vi "Motor sequence -- FGV.vi"(7 "Motor params":T2, 8 "error in (no error)":errorcluster, 10 "current position (in)":dbl, 11 "Action":T1=enum."Full step") -> (0 "error out":errorcluster, 3 "Data out":bool[](array[boolean]), 5 "current position (out)":dbl)   [LabVIEW 2020, in "GUI.lvlib"]
uses:
  GUI.lvlib
  <userlib>/_OpenG.lib/array/array.llb/openg_array.lvlib
  <userlib>/_OpenG.lib/array/array.llb/Reverse 2D Array (Boolean)__ogtk.vi
  Support/Motor parameters.ctl
  FGV states.ctl
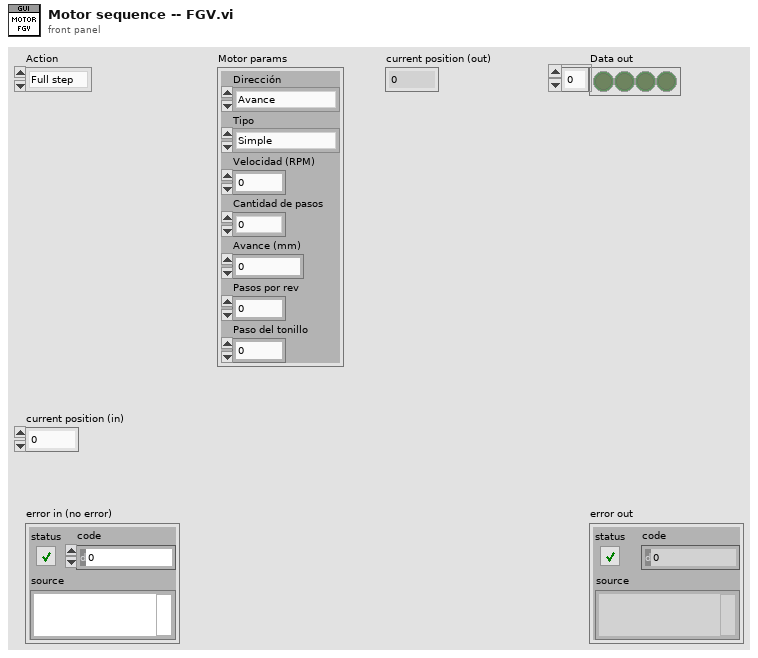
[diagram p1: front panel]
types:
  T1 = typedef "GUI.lvlib/FGV states.ctl" = enum16{"Read", "Full step", "Half step", "Release", "Reset"}
  T2 = typedef "GUI.lvlib/Motor parameters.ctl" = cluster{"Dirección":enum16{"Avance", "Retroceso"}, "Tipo":enum16{"Simple", "Medio paso"}, "Velocidad (RPM)":dbl, "Cantidad de pasos":i32, "Avance (mm)":dbl, "Pasos por rev":dbl, "Paso del tonillo":dbl}
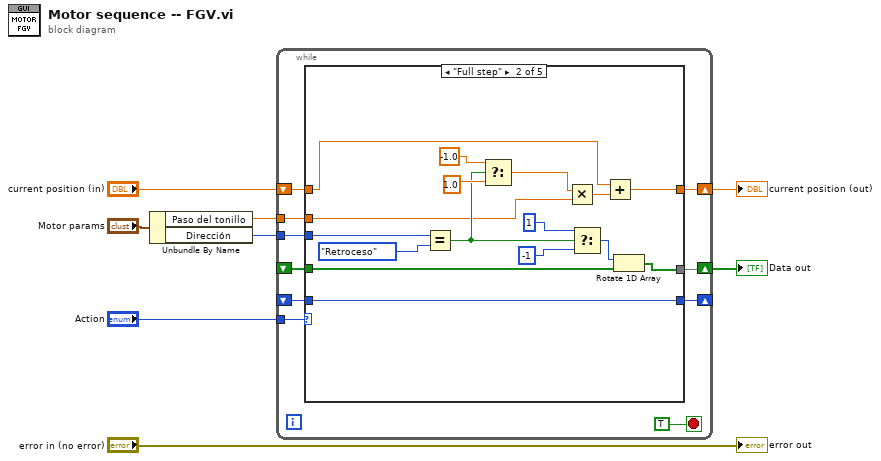
[diagram p0: block diagram]
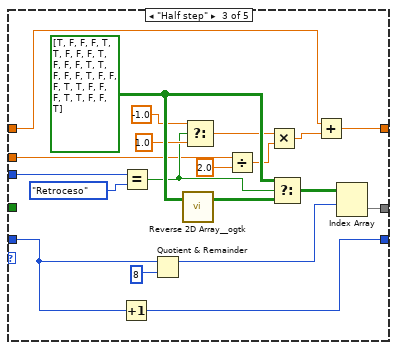
[diagram p3: hidden frame]
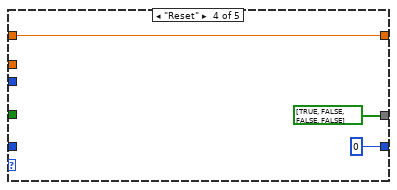
[diagram p4: hidden frame]
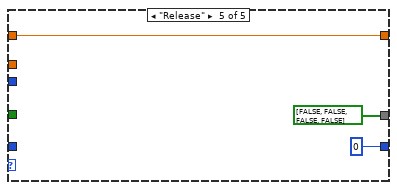
[diagram p5: hidden frame]
diagram:
  n1 = Unbundle By Name("Motor params") -> ("Paso del tonillo"=w2:dbl, "Dirección"=w5:enum16{"Avance", "Retroceso"})
  n2 = while {
    shift-right: [w16] -> w7
    shift-left: _ -> [w17]
    tunnel: w5 -> [w15]
    shift-right: [w13] -> _
    shift-left: _ -> [w14]
    shift-right: [w11] -> w3
    shift-left: "current position (in)" -> [w12]
    tunnel: w2 -> [w10]
    tunnel: "Action" -> [w9]
    stop <- TRUE stop-if-true
    n3 = case shown="\"Full step\"" w9 {
      tunnel: w17 -> [w21 w37 _ _ _]
      tunnel: [w21 w36 w56 bool[] [TRUE, FALSE, FALSE, FALSE] bool[] [FALSE, FALSE, FALSE, FALSE]] -> w16
      tunnel: w15 -> [_ w35 w53 _ _]
      tunnel: w14 -> [w20 w30 w50 _ _]
      tunnel: [w20 w30 w49 0 0] -> w13
      tunnel: w12 -> [w19 w24 w40 w58 w61]
      tunnel: [w19 w23 w41 w58 w61] -> w11
      tunnel: w10 -> [_ w25 w39 _ _]
      frame "Read", Default {
      }
      frame "Full step" {
        n4 = Equal?(x=w35, y=enum16{"Avance", "Retroceso"}."Retroceso") -> (x = y?=w27:bool)
        n5 = Select(t=-1.0 ("y"), s=w27, f=1.0 ("y")) -> (s? t:f=w22:dbl)
        n6 = Multiply(x=w22, y=w25) -> (x*y=w26:dbl)
        n7 = Select(t=1 ("n"), s=w27, f=-1 ("n")) -> (s? t:f=w31:i32)
        n8 = Add(x=w24, y=w26) -> (x+y=w23:dbl)
        n9 = Rotate 1D Array(1:w37, 2:w31) -> (0:w36:bool[])
      }
      frame "Half step" {
        w52 = bool[][] [[TRUE, FALSE, FALSE, FALSE], [TRUE, TRUE, FALSE, FALSE], [FALSE, TRUE, FALSE, FALSE], [FALSE, TRUE, TRUE, FALSE], [FALSE, FALSE, TRUE, FALSE], [FALSE, FALSE, TRUE, TRUE], [FALSE, FALSE, FALSE, TRUE], [TRUE, FALSE, FALSE, TRUE]]
        n10 = Increment(x=w50) -> (x+1=w49:i32)
        n11 = Equal?(x=w53, y=enum16{"Avance", "Retroceso"}."Retroceso") -> (x = y?=w45:bool)
        n12 = Quotient & Remainder(x=w50, y=8) -> (x-y*floor(x/y)=w55:i32)  [unwired: 1 out]
        n13 = call-poly <userlib>:"Reverse 2D Array__ogtk.vi"("Array"=w52) -> ("Reversed Array"=w51:bool[][])  [unwired: 2 in]
        n14 = Select(t=-1.0 ("y"), s=w45, f=1.0 ("y")) -> (s? t:f=w44:dbl)
        n15 = Divide(x=w39, y=2.0) -> (x/y=w38:dbl)
        n16 = Multiply(x=w44, y=w38) -> (x*y=w43:dbl)
        n17 = Select(t=w52, s=w45, f=w51) -> (s? t:f=w48:bool[][])
        n18 = Add(x=w40, y=w43) -> (x+y=w41:dbl)
        n19 = Index Array(array=w48, index (row)=w55) -> (element=w56:bool[])  [unwired: 1 in]
      }
      frame "Reset" {
      }
      frame "Release" {
      }
    }
  }
  "Data out" <- w7
  "current position (out)" <- w3
  "error out" <- "error in (no error)"
